vi "CallDialog.vi"(2 "vi name":string) -> ()   [LabVIEW 2015]
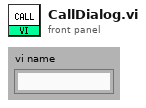
[diagram p1: front panel]
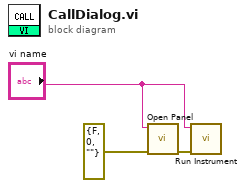
[diagram p0: block diagram]
diagram:
  n1 = call <vilib>:"Open Panel.vi"("error in (no error)"=errorcluster {"status"=FALSE, "code"=0, "source"=""}, "VI name"="vi name") -> ("error out"=w3:errorcluster)  [unwired: 1 in, 8 out]
  n2 = call <vilib>:"Run Instrument.vi"("error in (no error)"=w3, "VI name"="vi name") -> ()  [unwired: 10 out]
